vi "VS LAVA.vi"() -> ()   [LabVIEW 2017, in "LVJSON Tests.lvlib"]
uses:
  LVJSON Tests.lvlib
  <vilib>/addons/JSON API/JSON Object/JSON Object.lvclass
  <vilib>/addons/JSON API/JSON Scalar/JSON Scalar.lvclass
  C:/Program Files (x86)/National Instruments/LabVIEW 2017/vi.lib/addons/JSON API/JSON Value/JSON Value.lvclass
  JSON Data Classes/JSON Numeric/JSON Numeric.lvclass
  C:/Users/tblair/Documents/Git Projects/LVJSON/JSON Data Classes/JSON Datatype/JSON Datatype.lvclass
  <vilib>/addons/JSON API/JSON Scalar/Set DBL.vi
  JSON Data Classes/JSON Object/New JSON Object.vi
  JSON Data Classes/JSON Numeric/New JSON Numeric.vi
  JSON Data Classes/JSON Object/Insert Key Value Pair (Multi).vi
  JSON Data Classes/JSON Object/JSON Object.lvclass
  JSON Data Classes/JSON Datatype/JSON Datatype.lvclass
  <vilib>/addons/JSON API/Get Polymorphic/JSON GetSet.lvlib
  C:/Users/tblair/Documents/Git Projects/LVJSON/JSON Data Classes/JSON Basic Type/JSON Basic Type.lvclass
panel:
  out "lvjson generation faster?":bool
  out "generation ratio":dbl
  out "lvjson generation time":dbl
  out "i3 generation time":dbl
  out "unflatten ratio":dbl
  out "flatten ratio":dbl
  in  "# of elements":i32
  out "lvjson flatten faster?":bool
  out "lvjson unflatten faster?":bool
  out "LAVA String":string
  out "lvjson String":string
  out "lvjson unflatten time":dbl
  out "lvjson flatten time":dbl
  out "i3 unflatten time":dbl
  out "i3 flatten time":dbl
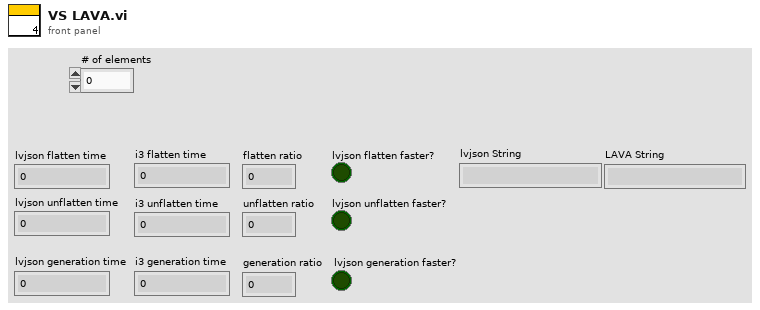
[diagram p1: front panel]
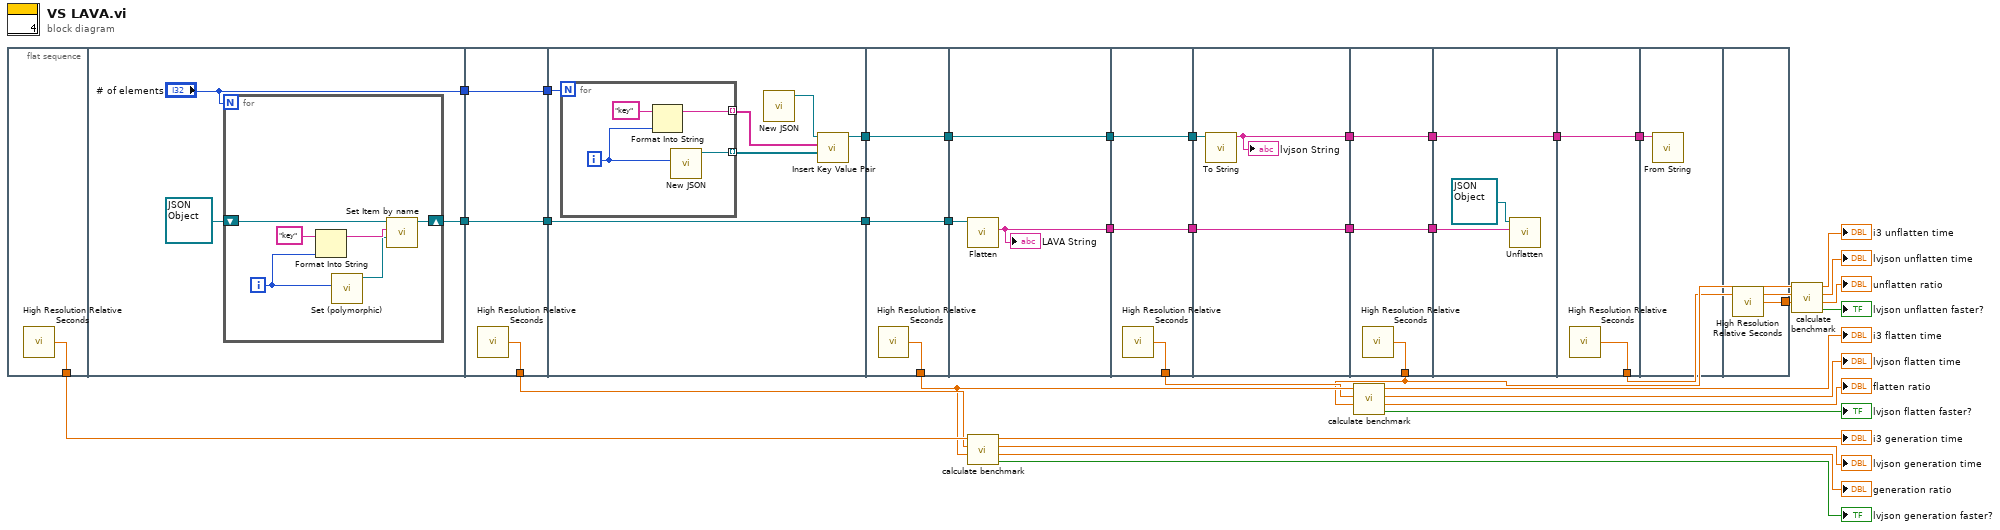
[diagram p0: block diagram]
diagram:
  n1 = flat-sequence {
    tunnel: [w38] -> w8
    tunnel: ["# of elements"] -> w29
    tunnel: [w40] -> w27
    tunnel: w29 -> [w50]
    tunnel: [w50] -> w28
    tunnel: w27 -> [w48]
    tunnel: [w49] -> w7
    tunnel: [w48] -> w23
    tunnel: w28 -> [w56]
    tunnel: w23 -> [w52]
    tunnel: [w52] -> w12
    tunnel: [w51] -> w10
    tunnel: w12 -> [w63]
    tunnel: [w63] -> w11
    tunnel: w10 -> [w62]
    tunnel: [w62] -> w9
    tunnel: [w61] -> w6
    tunnel: w11 -> [w65]
    tunnel: w9 -> [w66]
    tunnel: [w66] -> w22
    tunnel: [w64] -> w20
    tunnel: [w69] -> w5
    tunnel: w22 -> [w68]
    tunnel: [w68] -> w21
    tunnel: w20 -> [w67]
    tunnel: [w67] -> w19
    tunnel: w21 -> [w72]
    tunnel: w19 -> [w71]
    tunnel: [w71] -> w18
    tunnel: [w70] -> w16
    tunnel: [w75] -> w4
    tunnel: w18 -> [w74]
    tunnel: [w74] -> w17
    tunnel: w16 -> [w73]
    tunnel: [w73] -> w15
    tunnel: w17 -> [w77]
    tunnel: w15 -> [w78]
    tunnel: [w78] -> w14
    tunnel: [w80] -> w3
    tunnel: w14 -> [w79]
    tunnel: [w79] -> w13
    tunnel: w13 -> [w81]
    tunnel: [w82] -> w2
    frame #0 {
      n2 = call <vilib>:"High Resolution Relative Seconds.vi"() -> ("relative seconds"=w38:dbl)
    }
    frame #1 {
      n3 = for {
        N: "# of elements" -> [_]
        shift-right: [w43] -> w40
        shift-left: refnum<class "JSON Object.lvclass"> refnum ("JSON Object in") -> [w42]
        i -> [w44]
        n4 = Format Into String(initial string="key", w44) -> (resulting string=w46:string)  [unwired: 2 in, 1 out]
        n5 = call-poly <vilib>:"Set (polymorphic).vi"("Numeric"=w44) -> ("JSON Scalar out"=w45:refnum<class "JSON Scalar.lvclass">)  [unwired: 9 in, 1 out]
        n6 = call-dynamic "Set Item by name.vi"("Value"=w45, "name"=w46, "JSON Object in"=w42) -> ("JSON Object out"=w43:refnum<class "JSON Object.lvclass">)  [unwired: 6 in, 2 out]
      }
    }
    frame #2 {
      n7 = call <vilib>:"High Resolution Relative Seconds.vi"() -> ("relative seconds"=w49:dbl)
    }
    frame #3 {
      n8 = for {
        N: w56 -> [_]
        tunnel: [w59] -> w54 mode=indexing
        tunnel: [w57] -> w53 mode=indexing
        i -> [w58]
        n9 = Format Into String(initial string="key", w58) -> (resulting string=w59:string)  [unwired: 2 in, 1 out]
        n10 = call-poly "New JSON.vi"("value"=w58) -> ("JSON String out"=w57:refnum<class "JSON Numeric.lvclass">)  [unwired: 9 in, 1 out]
      }
      n11 = call-poly "New JSON.vi"() -> ("JSON Object out"=w55:refnum<class "JSON Object.lvclass">)  [unwired: 10 in, 1 out]
      n12 = call-poly "Insert Key Value Pair.vi"("values"=w53, "keys"=w54, "JSON Object in"=w55) -> ("JSON Object out"=w51:refnum<class "JSON Object.lvclass">)  [unwired: 7 in, 1 out]
    }
    frame #4 {
      n13 = call <vilib>:"High Resolution Relative Seconds.vi"() -> ("relative seconds"=w61:dbl)
    }
    frame #5 {
      n14 = call-dynamic "Flatten.vi"("JSON Object in"=w65) -> ("<JSON>"=w64:string)  [unwired: 9 in, 1 out]
      "LAVA String" <- w64
    }
    frame #6 {
      n15 = call <vilib>:"High Resolution Relative Seconds.vi"() -> ("relative seconds"=w69:dbl)
    }
    frame #7 {
      n16 = call-dynamic "To String.vi"("JSON Object in"=w72) -> ("String"=w70:string)  [unwired: 9 in, 1 out]
      "lvjson String" <- w70
    }
    frame #8 {
      n17 = call <vilib>:"High Resolution Relative Seconds.vi"() -> ("relative seconds"=w75:dbl)
    }
    frame #9 {
      n18 = call-dynamic "Unflatten.vi"("JSON stream"=w77, "JSON Object In"=refnum<class "JSON Object.lvclass"> refnum) -> ()  [unwired: 6 in, 4 out]
    }
    frame #10 {
      n19 = call <vilib>:"High Resolution Relative Seconds.vi"() -> ("relative seconds"=w80:dbl)
    }
    frame #11 {
      n20 = call "From String.vi"("JSON String"=w81) -> ()  [unwired: 9 in, 2 out]
    }
    frame #12 {
      n21 = call <vilib>:"High Resolution Relative Seconds.vi"() -> ("relative seconds"=w82:dbl)
    }
  }
  n22 = call "calculate benchmark.vi"("end"=w6, "middle"=w7, "beginning"=w8) -> ("lvjson faster?"=→"lvjson generation faster?":bool, "ratio"=→"generation ratio":dbl, "lvjson time"=→"lvjson generation time":dbl, "i3 time"=→"i3 generation time":dbl)  [unwired: 5 in]
  n23 = call "calculate benchmark.vi"("end"=w4, "middle"=w5, "beginning"=w6) -> ("lvjson faster?"=→"lvjson flatten faster?":bool, "ratio"=→"flatten ratio":dbl, "lvjson time"=→"lvjson flatten time":dbl, "i3 time"=→"i3 flatten time":dbl)  [unwired: 5 in]
  n24 = call "calculate benchmark.vi"("end"=w2, "middle"=w3, "beginning"=w4) -> ("lvjson faster?"=→"lvjson unflatten faster?":bool, "ratio"=→"unflatten ratio":dbl, "lvjson time"=→"lvjson unflatten time":dbl, "i3 time"=→"i3 unflatten time":dbl)  [unwired: 5 in]
